vi "load OME modify single node and save.vi"(7 "XML File Path":path, 10 "New Value (String)":string, 11 "XPath expression to node":string) -> (3 "XML string out":string)   [LabVIEW 2012]
doc: "SciScan 1.2 160622"
uses:
  <vilib>/xml/Close Reference(Node).vi
  <resource>/objmgr/DOMUserDefRef.rc
  <vilib>/xml/NI_XML.lvlib
panel:
  out "Parse Errors":string
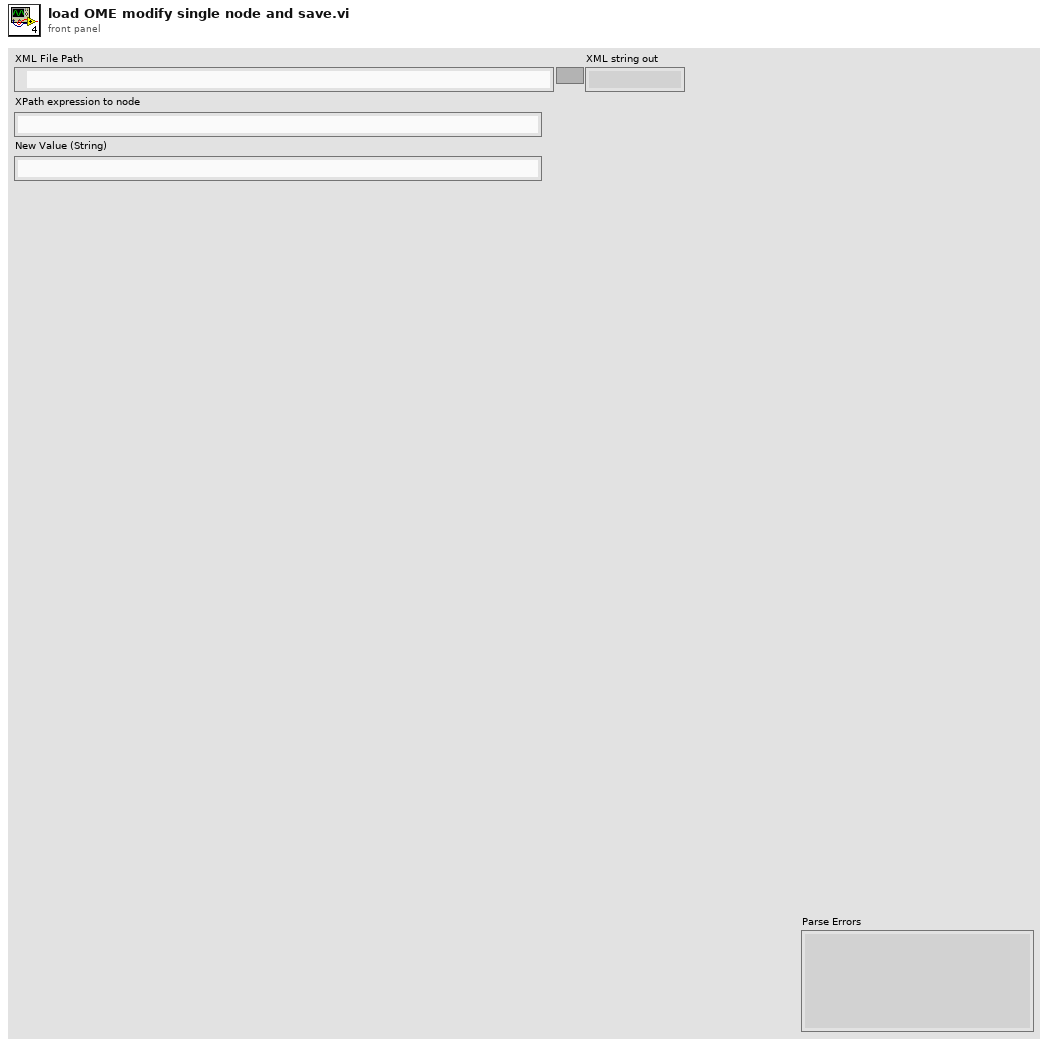
[diagram p1: front panel]
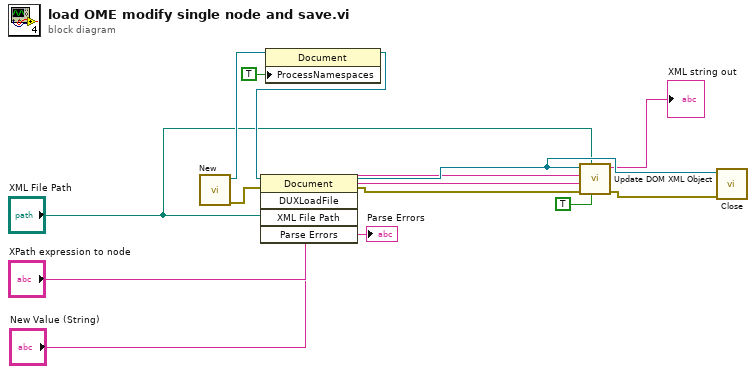
[diagram p0: block diagram]
diagram:
  n1 = call <vilib>:"New.vi"() -> ("error out"=w9:errorcluster, "DOM document out"=w12:refnum<k20>)  [unwired: 8 in]
  n2 = property class="Document"(reference=w12, "ProcessNamespaces"=TRUE ("Process Namespaces")) -> (reference out=w13:refnum<k20>)  [unwired: 1 in, 1 out]
  n3 = invoke class="Document" method="DUXLoadFile"(reference=w13, error in=w9, "XML File Path"="XML File Path") -> (reference out=w7:refnum<k20>, error out=w5:errorcluster, "Parse Errors"=→"Parse Errors":string)  [unwired: 2 in, 2 out]
  n4 = call "Update DOM XML Object.vi"("Write to File?"=TRUE, "XML File Path"="XML File Path", "error in (no error)"=w5, "New Value (String)"="New Value (String)", "XPath expression to node"="XPath expression to node", "DOM Refnum (XML Document)"=w7) -> ("error out"=w6:errorcluster, "XML string out"=→"XML string out":string)  [unwired: 4 in]
  n5 = call-poly <vilib>:"Close.vi"("error in (no error)"=w6, "node"=w7) -> ()  [unwired: 7 in, 1 out]
